vi "Vision Processor_modified.vi"(5 "error in":errorcluster, 7 "Image In":T2) -> (0 "error out":errorcluster, 3 "Image Out":T2(plugin-control))   [LabVIEW 2013]
uses:
  <vilib>/vision/Image Controls.llb/IMAQ Image.ctl
  <vilib>/vision/NI_Vision_Development_Module.lvlib
panel:
  in  "Green or Sat Range":cluster{"Lower value":i32, "Upper value":i32}={"Lower value"=128, "Upper value"=255}
  out "HSL Histogram":T1(graph)
  out "Image In":T2(plugin-control)
  # "0  center of mass x\n1  center of mass y\n2  first pixel x\n3  first pixel y\n4  bounding rect left\n5  bounding rect top\n6  bounding rect right\n7  bounding rect bottom\n8 max feret diameter start x\n9  max feret diameter start y\n10 max feret diameter end x\n11 max feret diameter end y\n12 max horiz segment length left\n13 max horiz segment length right\n14 max horiz segment length row\n15 bounding rect width \n16 bounding rect height\n17 bounding rect diagional\n..\n33 area"
  # "13'3\"\n3'9\""
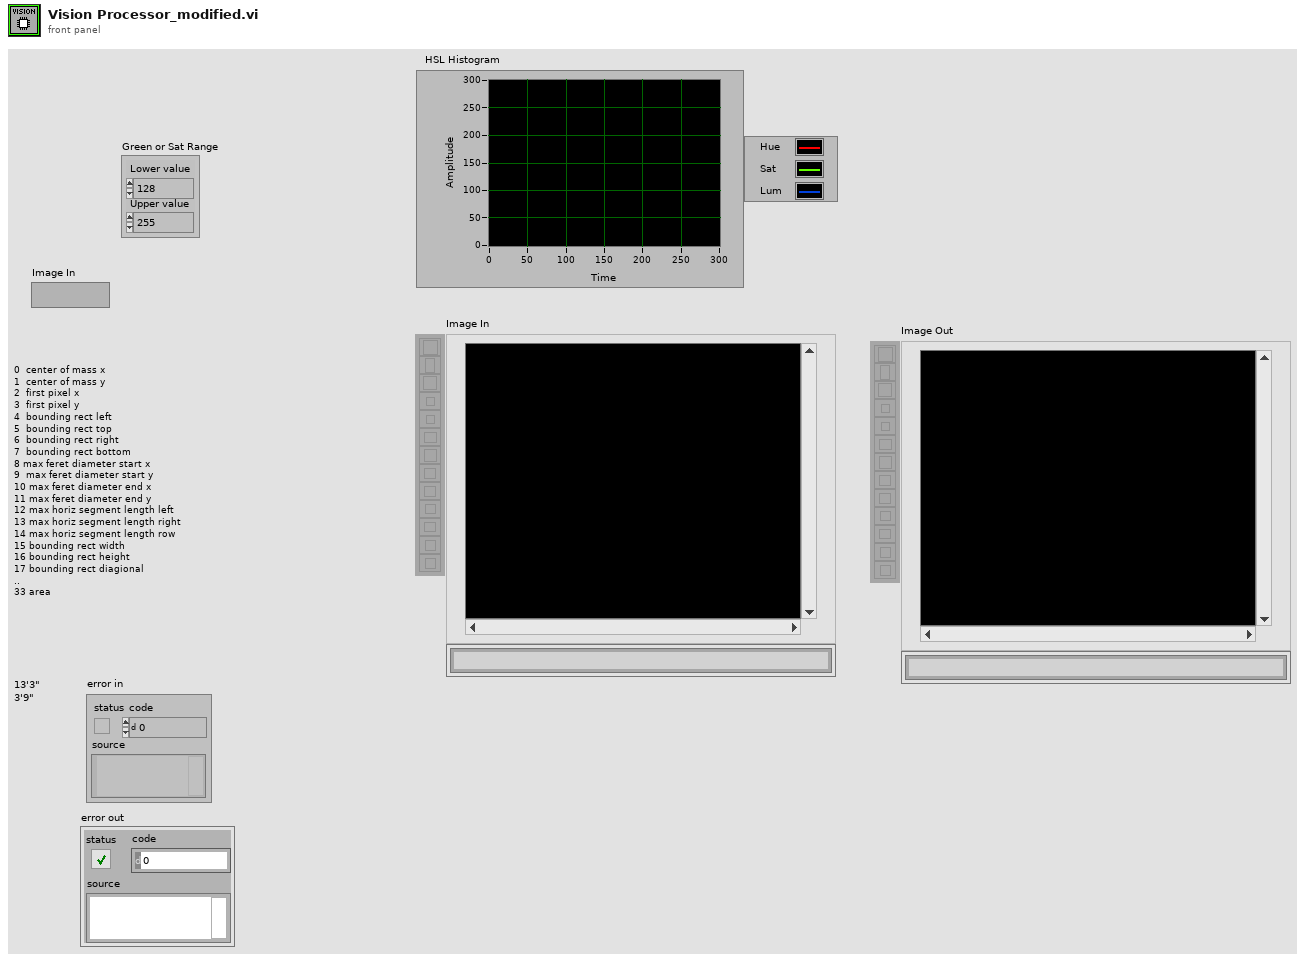
[diagram p1: front panel]
types:
  T1 = cluster{"Starting Value":sgl, "Incremental Value":sgl, "Histogram":u32[]}[]
  T2 = typedef "IMAQ Image.ctl" = refnum<image>
  T3 = enum32{"AutoM", "Close", "Dilate", "Erode", "Gradient", "Gradient out", "Gradient in", "Hit miss", "Open", "PClose", "POpen", "Thick", "Thin"}
  T4 = typedef "Image Type" = u32
  T5 = cluster{"Starting Value":sgl, "Incremental Value":sgl, "Histogram":u32[]}
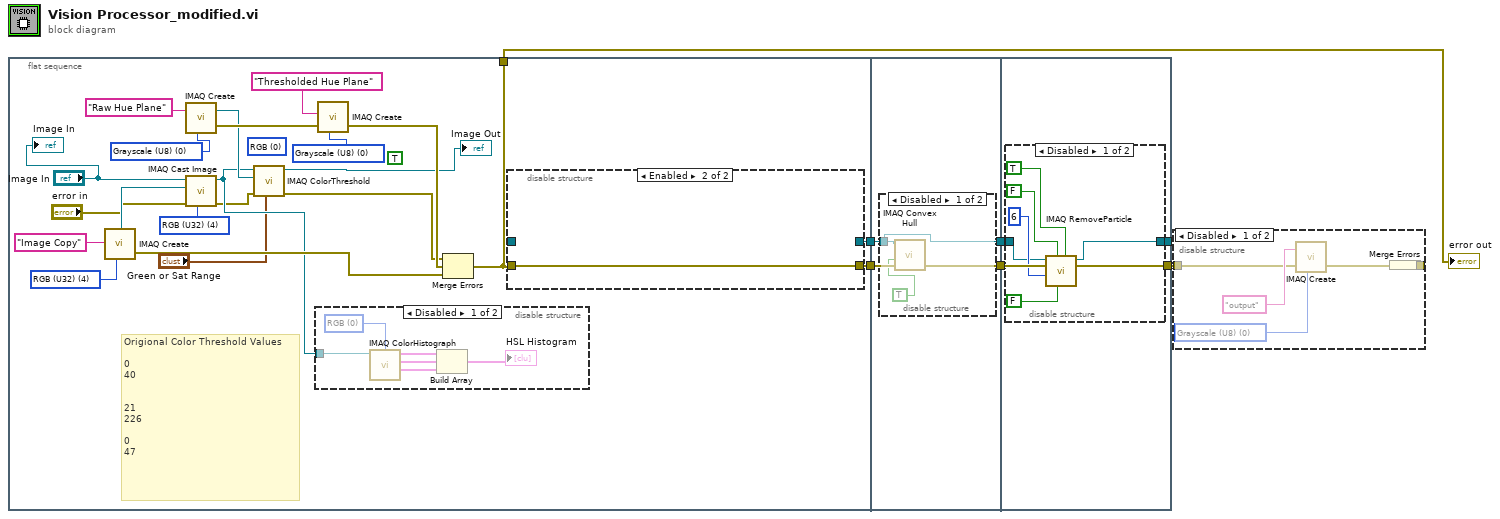
[diagram p0: block diagram]
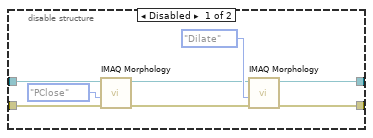
[diagram p4: hidden frame]
diagram:
  n1 = flat-sequence {
    tunnel: [w26] -> w6
    tunnel: [w25] -> w5
    tunnel: [w8] -> w1
    tunnel: w6 -> [w44]
    tunnel: w5 -> [w45]
    tunnel: [w44] -> w4
    tunnel: [w45] -> w3
    tunnel: [w48] -> _
    tunnel: w4 -> [w49]
    tunnel: w3 -> [w50]
    tunnel: [w50] -> w2
    frame #0 {
      (unwired) TRUE ("Keep/Replace Value (Replace)")
      (unwired) u16 0 items=["RGB", "HSL", "HSV", "HSI"] ("Color Mode")
      w19 = T4 0 items=["Grayscale (U8)", "Grayscale (I16)", "Grayscale (SGL)", "Complex (CSG)", "RGB (U32)", "HSL (U32)", "RGB (U64)", "Grayscale (U16)"] ("Image Type")
      w21 = T4 0 items=["Grayscale (U8)", "Grayscale (I16)", "Grayscale (SGL)", "Complex (CSG)", "RGB (U32)", "HSL (U32)", "RGB (U64)", "Grayscale (U16)"] ("Image Type")
      w23 = T4 4 items=["Grayscale (U8)", "Grayscale (I16)", "Grayscale (SGL)", "Complex (CSG)", "RGB (U32)", "HSL (U32)", "RGB (U64)", "Grayscale (U16)"] ("Image Type")
      w27 = T4 4 items=["Grayscale (U8)", "Grayscale (I16)", "Grayscale (SGL)", "Complex (CSG)", "RGB (U32)", "HSL (U32)", "RGB (U64)", "Grayscale (U16)"] ("Image Type")
      # "Origional Color Threshold Values\n\n0\n40\n\n\n21\n226\n\n0\n47"
      n2 = call "IMAQ Create"("Image Name"="Image Copy", "Image Type"=w27) -> ("New Image"=w16:T2, "error out"=w24:errorcluster)  [unwired: 3 in]
      n3 = call "IMAQ Create"("Image Name"="Raw Hue Plane", "Image Type"=w21) -> ("New Image"=w13:T2, "error out"=w18:errorcluster)  [unwired: 3 in]
      n4 = call "IMAQ Cast Image"("Image Type"=w23, "error in (no error)"="error in", "Image Dst"=w16, "Image Src"="Image In") -> ("error out"=w10:errorcluster, "Image Dst Out"=w12:T2)  [unwired: 6 in]
      n5 = call "IMAQ ColorThreshold"("Green or Sat Range"="Green or Sat Range", "error in (no error)"=w10, "Image Dst"=w13, "Image Src"=w12) -> ("error out"=w7:errorcluster, "Image Dst Out"=→"Image Out":T2)  [unwired: 6 in]
      n6 = disable-structure shown="Disabled" {
        disable-tunnel: w12 -> [w29 _]
        frame Disabled {
          w30 = u16 0 items=["RGB", "HSL", "HSV", "HSI"] ("Color Mode")
          n7 = call "IMAQ ColorHistograph"("Color Mode"=w30, "Image Src"=w29) -> ("Red or Hue Histogram Graph"=w34:T5, "Green or Sat Histogram Graph"=w33:T5, "Blue or Luma or Val or Inten Histogram Graph"=w32:T5)  [unwired: 4 in, 1 out]
          n8 = Build Array(w34, w33, w32) -> (→"HSL Histogram":T1)
        }
        frame Enabled {
        }
      }
      n9 = call "IMAQ Create"("Image Name"="Thresholded Hue Plane", "Image Type"=w19, "error in (no error)"=w18) -> ("error out"=w17:errorcluster)  [unwired: 2 in, 1 out]
      n10 = Merge Errors(w7, w17, w24) -> (w8:errorcluster)
      n11 = disable-structure shown="Enabled" {
        disable-tunnel: _ -> [w41 _]
        disable-tunnel: w8 -> [w40 w43]
        disable-tunnel: [w36 _] -> w26
        disable-tunnel: [w35 w43] -> w25
        frame Disabled {
          n12 = call "IMAQ Morphology"("error in (no error)"=w40, "Operation"=T3."PClose", "Image Src"=w41) -> ("error out"=w38:errorcluster, "Image Dst Out"=w37:T2)  [unwired: 7 in]
          n13 = call "IMAQ Morphology"("error in (no error)"=w38, "Operation"=T3."Dilate", "Image Src"=w37) -> ("error out"=w35:errorcluster, "Image Dst Out"=w36:T2)  [unwired: 7 in]
        }
        frame Enabled {
        }
      }
      "Image In" <- "Image In"
    }
    frame #1 {
      n14 = disable-structure shown="Disabled" {
        disable-tunnel: w44 -> [w46 _]
        frame Disabled {
          n15 = call "IMAQ Convex Hull"("Connectivity 4/8 (8)"=TRUE, "Image Src"=w46) -> ()  [unwired: 2 in, 8 out]
        }
        frame Enabled {
        }
      }
    }
    frame #2 {
      n16 = disable-structure shown="Disabled" {
        disable-tunnel: w49 -> [w52 _]
        disable-tunnel: [w51 _] -> w48
        frame Disabled {
          n17 = call "IMAQ RemoveParticle"("Connectivity 4/8 (8)"=TRUE, "Low Pass/High Pass (Low)"=FALSE, "Square/Hexa (Square)"=FALSE, "Number of Erosion"=6, "Image Src"=w52) -> ("Image Dst Out"=w51:T2)  [unwired: 2 in, 4 out]
        }
        frame Enabled {
        }
      }
    }
  }
  n18 = disable-structure shown="Disabled" {
    disable-tunnel: [w58 _] -> _
    disable-tunnel: w2 -> [w57 _]
    frame Disabled {
      w61 = T4 0 items=["Grayscale (U8)", "Grayscale (I16)", "Grayscale (SGL)", "Complex (CSG)", "RGB (U32)", "HSL (U32)", "RGB (U64)", "Grayscale (U16)"] ("Image Type")
      n19 = call "IMAQ Create"("Image Name"="output", "Image Type"=w61, "error in (no error)"=w57) -> ("error out"=w59:errorcluster)  [unwired: 2 in, 1 out]
      n20 = Merge Errors(w59) -> (w58:errorcluster)
    }
    frame Enabled {
    }
  }
  "error out" <- w1
